vi "Image Type.vi"(8 "error in (no error)":errorcluster, 10 "Image Type":enum16{"<Select>", "TIFF", "RAW"}(ring), 11 "Controller in":refnum<class "Controller.lvclass">) -> (0 "error out":errorcluster, 3 "Controller out":refnum<class "Controller.lvclass">)   [LabVIEW 2022 SP3, in "Controller.lvlib" / "Controller.lvclass"]
uses:
  Controller.lvclass
  Controller.lvclass/Controller.ctl
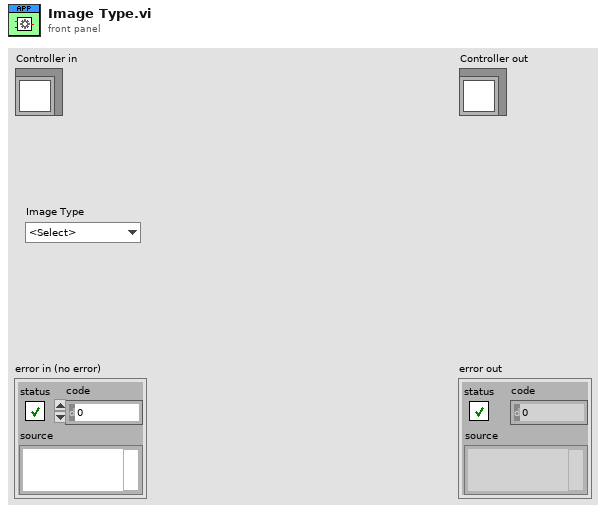
[diagram p1: front panel]
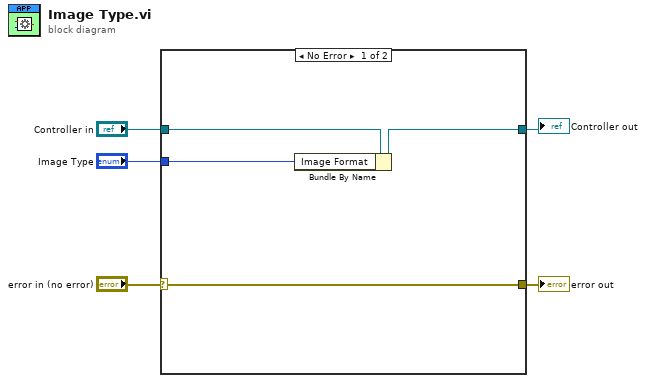
[diagram p0: block diagram]
diagram:
  n1 = case shown="No Error" "error in (no error)" {
    selector: "error in (no error)" -> [w6 w11]
    tunnel: "Controller in" -> [w9 w10]
    tunnel: [w8 w10] -> w4
    tunnel: "Image Type" -> [w7 _]
    tunnel: [w6 w11] -> w1
    frame No Error {
      n2 = Bundle By Name(cluster=w9, "Image Format"=w7) -> (w8:refnum<class "Controller.lvclass">)
    }
    frame Error {
    }
  }
  "error out" <- w1
  "Controller out" <- w4
